vi "SN Analyze.vi"(0 "Run Screen SN":string, 5 "Specified SNs":string[](array[string]), 9 "Data":string[][](array[string]), 11 "Profile":string[][](array[string])) -> (4 "Next SN":string, 8 "Untested SNs":string[](array[string]), 15 "Tested SNs":string[](array[string]))   [LabVIEW 2013]
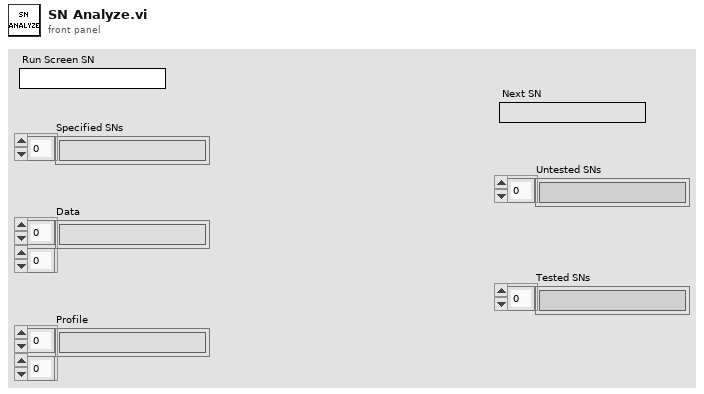
[diagram p1: front panel]
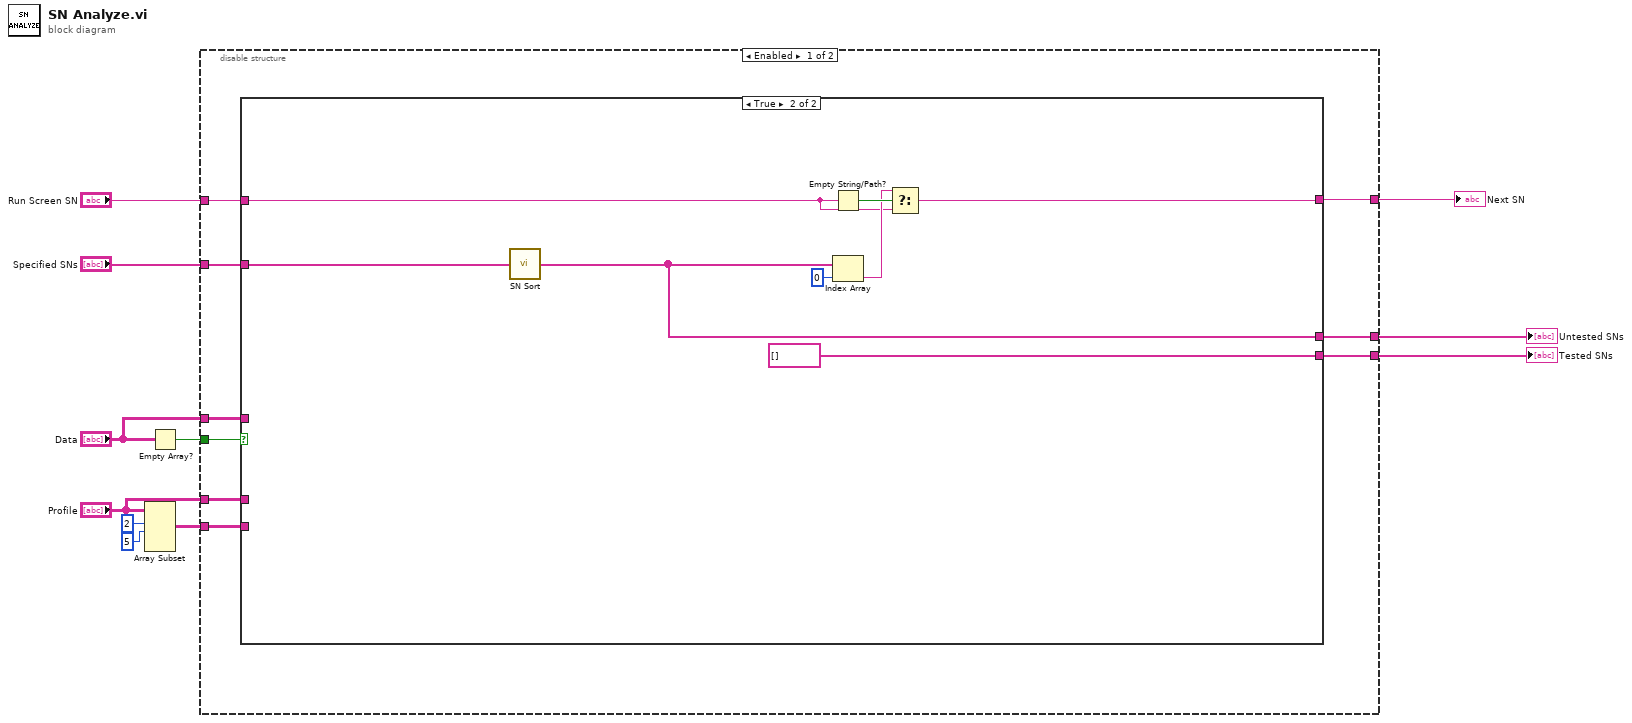
[diagram p0: block diagram]
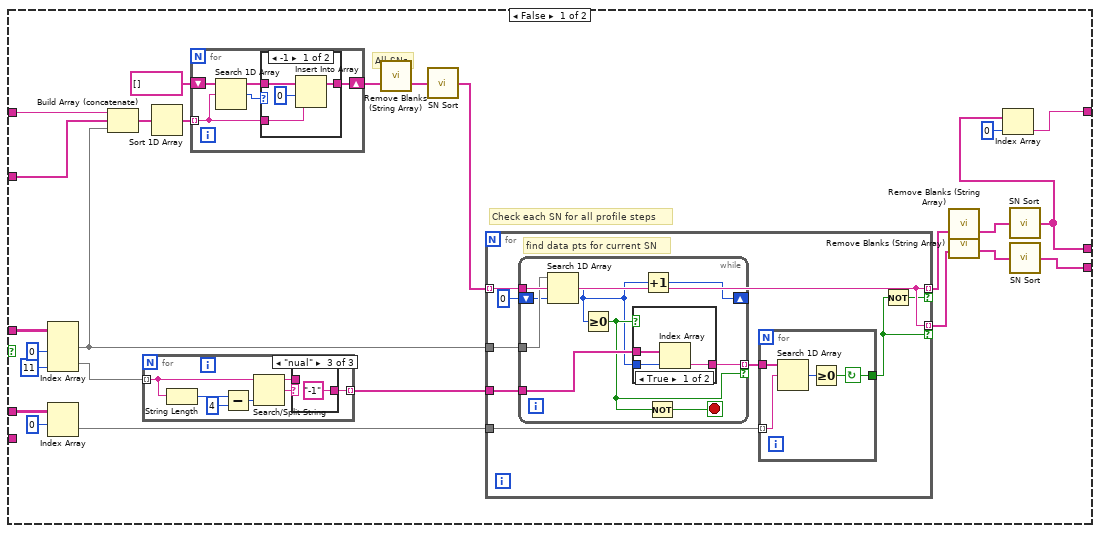
[diagram p2: hidden frame]
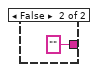
[diagram p5: hidden frame]
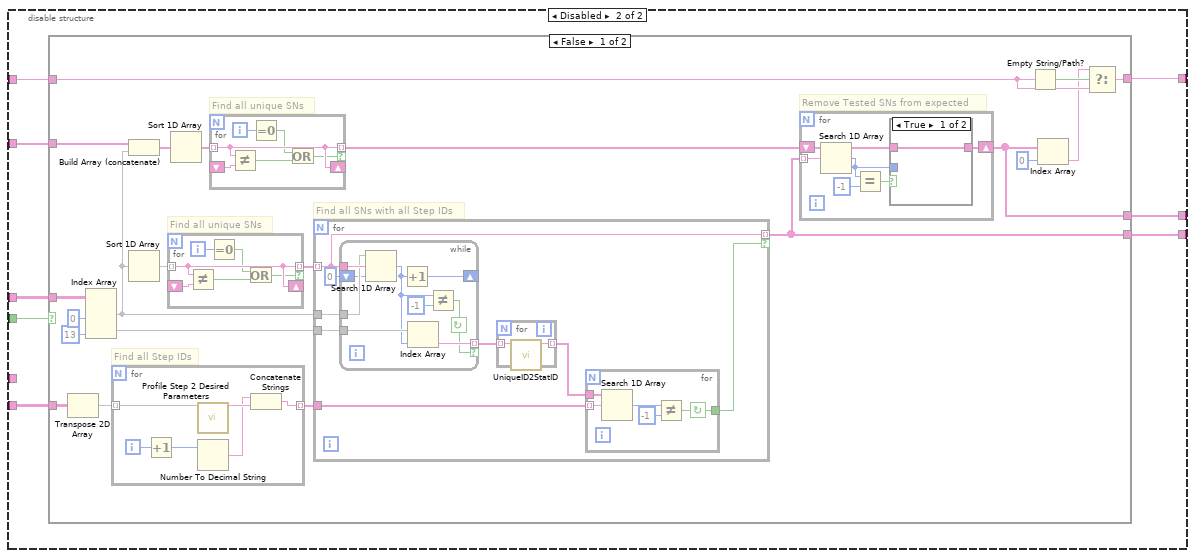
[diagram p7: hidden frame]
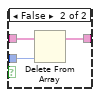
[diagram p8: hidden frame]
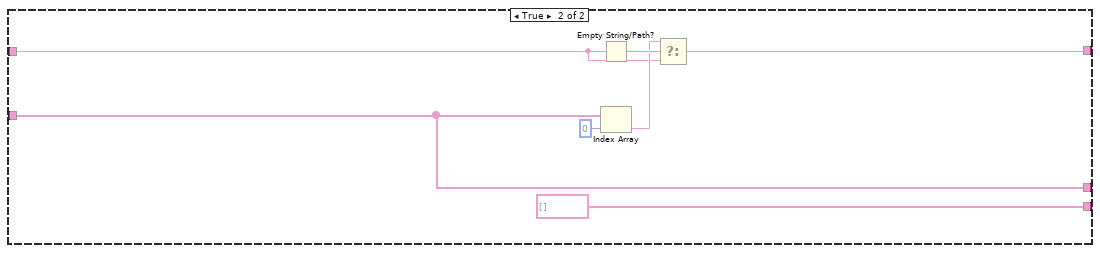
[diagram p9: hidden frame]
diagram:
  n1 = Array Subset(array="Profile", index (row)=2 ("index"), length (row)=5 ("length")) -> (w4:string[][])  [unwired: 2 in]
  n2 = Empty Array?(array="Data") -> (empty?=w11:bool)
  n3 = disable-structure shown="Enabled" {
    disable-tunnel: w11 -> [w20 w105]
    disable-tunnel: "Specified SNs" -> [w19 w104]
    disable-tunnel: "Run Screen SN" -> [w18 w103]
    disable-tunnel: [w17 w102] -> w8
    disable-tunnel: "Data" -> [w16 w101]
    disable-tunnel: [w15 w100] -> w1
    disable-tunnel: [w14 w99] -> w2
    disable-tunnel: w4 -> [w13 w98]
    disable-tunnel: "Profile" -> [w12 _]
    frame Enabled {
      n4 = case shown="True" w20 {
        tunnel: w19 -> [w42 w91]
        tunnel: w18 -> [w43 w92]
        tunnel: [w21 w93] -> w17
        tunnel: [w23 w90] -> w14
        tunnel: [w24 string[] [] ("Tested SNs")] -> w15
        tunnel: w13 -> [_ _]
        tunnel: w16 -> [w45 _]
        tunnel: w12 -> [w36 _]
        frame False {
          # "Check each SN for all profile steps"
          # "All SNs"
          n5 = Index Array(array=w45, index (col) #1=0 ("disabled index (col)"), index (col) #2=11 ("index (col)")) -> (element #1=w32:string[], element #2=w30:string[])  [unwired: 2 in]
          n6 = Index Array(array=w36, index (row)=0) -> (element=w31:string[])  [unwired: 1 in]
          n7 = Build Array (concatenate)(w43, w42, w32) -> (w41:string[])
          n8 = for {
            tunnel: w30 -> [w47] mode=indexing
            tunnel: [w46] -> w29 mode=indexing
            n9 = String Length(string=w47) -> (length=w48:i32)
            n10 = Subtract(x=w48, y=4) -> (x-y=w51:i32)
            n11 = Search/Split String(string=w47, offset (0)=w51) -> (substring before match=w52:string, match + rest of string=w50:string)  [unwired: 1 in, 1 out]
            n12 = case shown="\"nual\"" w50 {
              selector: w50 -> [w53 _ _]
              tunnel: [w53 w54 "-1"] -> w46
              tunnel: w52 -> [_ w54 _]
              frame Default {
              }
              frame " (M)" {
              }
              frame "nual" {
              }
            }
          }
          n13 = Sort 1D Array(array=w41) -> (sorted array=w40:string[])
          n14 = for {
            tunnel: w40 -> [w82] mode=indexing
            shift-right: [w81] -> w38
            shift-left: string[] [] ("sorted array") -> [w83]
            n15 = Search 1D Array(1D array=w83, element=w82) -> (index of element=w84:i32)  [unwired: 1 in]
            n16 = case shown="-1" w84 {
              tunnel: w83 -> [w88 w89]
              tunnel: w82 -> [w85 _]
              tunnel: [w87 w89] -> w81
              frame -1 {
                n17 = Insert Into Array(array=w88, index=0, new element=w85) -> (w87:string[])
              }
              frame Default {
              }
            }
          }
          n18 = call "Remove Blanks (String Array).vi"("Array In"=w38) -> ("Array Out"=w37:string[])  [unwired: 18 in]
          n19 = call "SN Sort.vi"("Array In"=w37) -> ("Array Out"=w33:string[])  [unwired: 14 in]
          n20 = for {
            tunnel: w33 -> [w58] mode=indexing
            tunnel: w32 -> [w63]
            tunnel: w29 -> [w62]
            tunnel: w31 -> [w60]
            tunnel: [w58] -> w26 mode=indexing if=w57
            tunnel: [w58] -> w25 mode=indexing if=w56
            # "find data pts for current SN"
            n21 = while {
              tunnel: w58 -> [w75]
              tunnel: w63 -> [w76]
              tunnel: w62 -> [w73]
              shift-right: [w68] -> _
              shift-left: 0 ("index of element") -> [w74]
              tunnel: [w72] -> w59 mode=indexing if=w71
              stop <- w70 stop-if-true
              n22 = Search 1D Array(1D array=w76, element=w75, start index (0)=w74) -> (index of element=w69:i32)
              n23 = Greater Or Equal To 0?(x=w69) -> (x >= 0?=w71:bool)
              n24 = case shown="True" w71 {
                tunnel: w73 -> [w79 _]
                tunnel: w69 -> [w78 _]
                tunnel: [w77 ""] -> w72
                frame True {
                  n25 = Index Array(array=w79, index=w78) -> (element=w77:string)
                }
                frame False {
                }
              }
              n26 = Increment(x=w69) -> (x+1=w68:i32)
              n27 = Not(x=w71) -> (.not. x?=w70:bool)
            }
            n28 = for {
              tunnel: w60 -> [w66] mode=indexing
              tunnel: w59 -> [w67]
              tunnel: [w64] -> w56
              stop <- w64 continue-if-true
              n29 = Search 1D Array(1D array=w67, element=w66) -> (index of element=w65:i32)  [unwired: 1 in]
              n30 = Greater Or Equal To 0?(x=w65) -> (x >= 0?=w64:bool)
            }
            n31 = Not(x=w56) -> (.not. x?=w57:bool)
          }
          n32 = call "Remove Blanks (String Array).vi"("Array In"=w26) -> ("Array Out"=w28:string[])  [unwired: 18 in]
          n33 = call "Remove Blanks (String Array).vi"("Array In"=w25) -> ("Array Out"=w27:string[])  [unwired: 18 in]
          n34 = call "SN Sort.vi"("Array In"=w28) -> ("Array Out"=w23:string[])  [unwired: 14 in]
          n35 = Index Array(array=w23, index=0) -> (element=w21:string)
          n36 = call "SN Sort.vi"("Array In"=w27) -> ("Array Out"=w24:string[])  [unwired: 14 in]
        }
        frame True {
          n37 = call "SN Sort.vi"("Array In"=w91) -> ("Array Out"=w90:string[])  [unwired: 14 in]
          n38 = Empty String/Path?(string/path=w92) -> (empty?=w96:bool)
          n39 = Index Array(array=w90, index=0) -> (element=w95:string)
          n40 = Select(t=w95, s=w96, f=w92) -> (s? t:f=w93:string)
        }
      }
    }
    frame Disabled {
      n41 = case shown="False" w105 {
        tunnel: w104 -> [w116 w181]
        tunnel: w103 -> [w110 w179]
        tunnel: [w109 w180] -> w102
        tunnel: [w111 w181] -> w99
        tunnel: [w112 string[] [] ("Tested SNs")] -> w100
        tunnel: w98 -> [w126 _]
        tunnel: w101 -> [w124 _]
        frame False {
          # "Remove Tested SNs from expected"
          # "Find all unique SNs"
          # "Find all SNs with all Step IDs"
          # "Find all Step IDs"
          # "Find all unique SNs"
          n42 = Transpose 2D Array(2D array=w126) -> (transposed array=w125:string[][])
          n43 = Index Array(array=w124, index (col) #1=0 ("disabled index (col)"), index (col) #2=13 ("index (col)")) -> (element #1=w117:string[], element #2=w121:string[])  [unwired: 2 in]
          n44 = for {
            tunnel: w125 -> [w178] mode=indexing
            tunnel: [w177] -> w118 mode=indexing
            i -> [w176]
            n45 = Increment(x=w176) -> (x+1=w175:i32)
            n46 = call "Profile Step 2 Desired Parameters.vi"("ProfileStep"=w178) -> ("ParameterSet"=w174:string)  [unwired: 14 in]
            n47 = Number To Decimal String(number=w175) -> (decimal integer string=w173:string)  [unwired: 1 in]
            n48 = Concatenate Strings(w173, w174) -> (w177:string)
          }
          n49 = Build Array (concatenate)(w116, w117) -> (w114:string[])
          n50 = Sort 1D Array(array=w117) -> (sorted array=w120:string[])
          n51 = for {
            tunnel: w120 -> [w147] mode=indexing
            shift-right: [w147] -> _
            shift-left: _ -> [w148]
            tunnel: [w147] -> w119 mode=indexing if=w145
            i -> [w146]
            n52 = Not Equal?(x=w147, y=w148) -> (x != y?=w144:bool)
            n53 = Equal To 0?(x=w146) -> (x = 0?=w143:bool)
            n54 = Or(x=w143, y=w144) -> (x .or. y?=w145:bool)
          }
          n55 = Sort 1D Array(array=w114) -> (sorted array=w115:string[])
          n56 = for {
            tunnel: w115 -> [w141] mode=indexing
            shift-right: [w141] -> _
            shift-left: _ -> [w142]
            tunnel: [w141] -> w113 mode=indexing if=w139
            i -> [w140]
            n57 = Not Equal?(x=w141, y=w142) -> (x != y?=w138:bool)
            n58 = Equal To 0?(x=w140) -> (x = 0?=w137:bool)
            n59 = Or(x=w137, y=w138) -> (x .or. y?=w139:bool)
          }
          n60 = for {
            tunnel: w117 -> [w156]
            tunnel: w121 -> [w155]
            tunnel: w119 -> [w152] mode=indexing
            tunnel: w118 -> [w153]
            tunnel: [w152] -> w112 mode=indexing if=w151
            n61 = while {
              tunnel: w152 -> [w172]
              tunnel: w156 -> [w171]
              tunnel: w155 -> [w168]
              shift-right: [w164] -> _
              shift-left: 0 -> [w170]
              tunnel: [w167] -> w150 mode=indexing if=w166
              stop <- w166 continue-if-true
              n62 = Search 1D Array(1D array=w171, element=w172, start index (0)=w170) -> (index of element=w165:i32)
              n63 = Increment(x=w165) -> (x+1=w164:i32)
              n64 = Index Array(array=w168, index=w165) -> (element=w167:string)
              n65 = Not Equal?(x=w165, y=-1) -> (x != y?=w166:bool)
            }
            n66 = for {
              tunnel: w150 -> [w158] mode=indexing
              tunnel: [w157] -> w149 mode=indexing
              n67 = call "UniqueID2StatID.vi"("UniqueID"=w158) -> ("ParameterSet"=w157:string)  [unwired: 10 in]
            }
            n68 = for {
              tunnel: w153 -> [w162] mode=indexing
              tunnel: w149 -> [w163]
              tunnel: [w159] -> w151
              stop <- w159 continue-if-true
              n69 = Search 1D Array(1D array=w163, element=w162) -> (index of element=w161:i32)  [unwired: 1 in]
              n70 = Not Equal?(x=w161, y=-1) -> (x != y?=w159:bool)
            }
          }
          n71 = for {
            tunnel: w112 -> [w132] mode=indexing
            shift-right: [w128] -> w111
            shift-left: w113 -> [w130]
            n72 = Search 1D Array(1D array=w130, element=w132) -> (index of element=w127:i32)  [unwired: 1 in]
            n73 = Equal?(x=w127, y=-1) -> (x = y?=w129:bool)
            n74 = case shown="True" w129 {
              tunnel: w130 -> [w133 w136]
              tunnel: [w133 w135] -> w128
              tunnel: w127 -> [_ w134]
              frame True {
              }
              frame False {
                n75 = Delete From Array(array=w136, index=w134) -> (array with subset deleted=w135:string[])  [unwired: 1 in, 1 out]
              }
            }
          }
          n76 = Empty String/Path?(string/path=w110) -> (empty?=w108:bool)
          n77 = Index Array(array=w111, index=0) -> (element=w107:string)
          n78 = Select(t=w107, s=w108, f=w110) -> (s? t:f=w109:string)
        }
        frame True {
          n79 = Empty String/Path?(string/path=w179) -> (empty?=w184:bool)
          n80 = Index Array(array=w181, index=0) -> (element=w183:string)
          n81 = Select(t=w183, s=w184, f=w179) -> (s? t:f=w180:string)
        }
      }
    }
  }
  "Tested SNs" <- w1
  "Untested SNs" <- w2
  "Next SN" <- w8
